vi "Table View.vi"(9 "Table":string[][](table)) -> ()   [LabVIEW 2018]
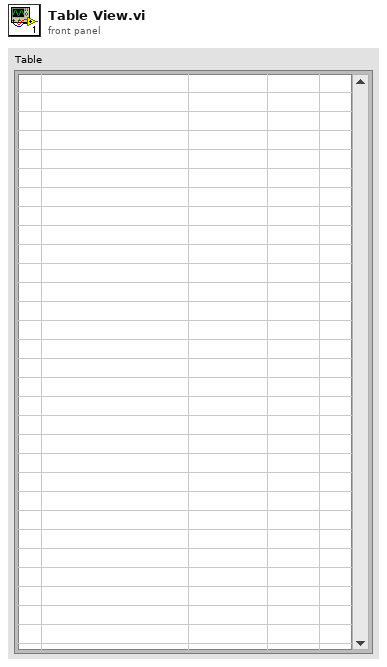
[diagram p1: front panel]
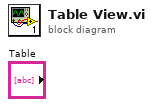
[diagram p0: block diagram]
diagram:
